vi "oax_Generate Amplitude Modulated Signal.vi"(7 "fs":dbl, 9 "envelop config":T1={"f"=0.4, "high limit"=8.0, "low limit"=1.0} {"low limit" format="%.2f"; "high limit" format="%.2f"; "f" format="%.2f"}, 10 "AM selection":u16(ring) items=["None", "Sine", "Triangle"], 11 "x":dbl[](array[numeric])) -> (3 "AM modulated signal":dbl[](array[numeric]))   [LabVIEW 2017]
uses:
  <vilib>/Analysis/NI_AALBase.lvlib
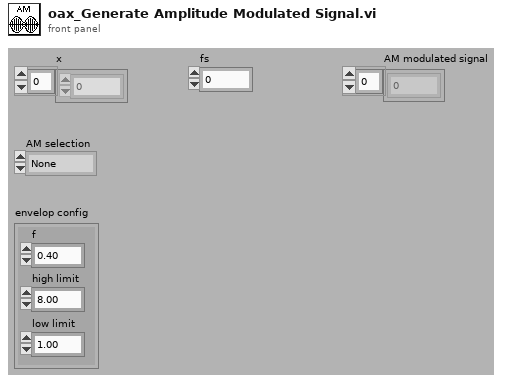
[diagram p1: front panel]
types:
  T1 = cluster{"f":dbl, "high limit":dbl, "low limit":dbl}
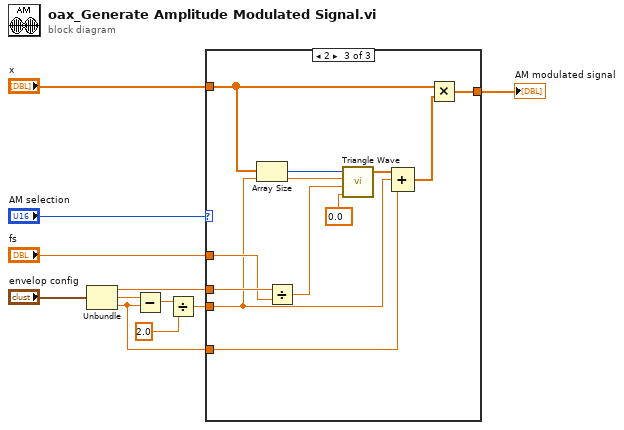
[diagram p0: block diagram]
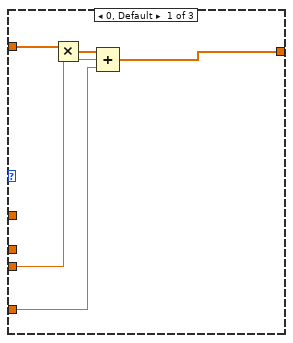
[diagram p2: hidden frame]
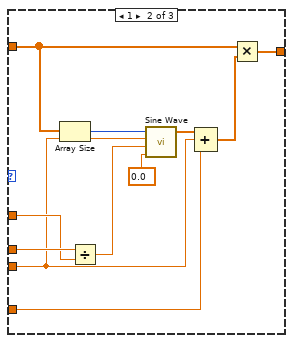
[diagram p3: hidden frame]
diagram:
  n1 = Unbundle("envelop config") -> ("f"=w2:dbl, "high limit"=w8:dbl, "low limit"=w4:dbl)
  n2 = Subtract(x=w8, y=w4) -> (x-y=w7:dbl)
  n3 = Divide(x=w7, y=2.0) -> (x/y=w5:dbl)
  n4 = case shown="2" "AM selection" {
    tunnel: "x" -> [w16 w20 w31]
    tunnel: w5 -> [w12 w17 w28]
    tunnel: w4 -> [w13 w21 w32]
    tunnel: [w14 w18 w29] -> w3
    tunnel: w2 -> [_ w25 w36]
    tunnel: "fs" -> [_ w24 w35]
    frame 0, Default {
      n5 = Multiply(x=w16, y=w12) -> (x*y=w15:dbl[])
      n6 = Compound Arithmetic op=ADD(w15, w12, w13) -> (w14:dbl[])
    }
    frame 1 {
      n7 = Array Size(array=w20) -> (size(s)=w26:i32)
      n8 = Divide(x=w25, y=w24) -> (x/y=w22:dbl)
      n9 = call <vilib>:"Sine Wave.vi"("samples"=w26, "amplitude"=w17, "frequency"=w22, "phase in"=0.0) -> ("sine wave"=w23:dbl[])  [unwired: 1 in, 2 out]
      n10 = Compound Arithmetic op=ADD(w23, w17, w21) -> (w19:dbl[])
      n11 = Multiply(x=w20, y=w19) -> (x*y=w18:dbl[])
    }
    frame 2 {
      n12 = Array Size(array=w31) -> (size(s)=w37:i32)
      n13 = Divide(x=w36, y=w35) -> (x/y=w33:dbl)
      n14 = call <vilib>:"Triangle Wave.vi"("samples"=w37, "amplitude"=w28, "frequency"=w33, "phase in"=0.0) -> ("triangle wave"=w34:dbl[])  [unwired: 1 in, 2 out]
      n15 = Compound Arithmetic op=ADD(w34, w28, w32) -> (w30:dbl[])
      n16 = Multiply(x=w31, y=w30) -> (x*y=w29:dbl[])
    }
  }
  "AM modulated signal" <- w3
